vi "Write Data to Log File.vi"(8 "Error In":errorcluster, 10 "queue out":refnum<queue>, 11 "Byte Stream File in":refnum<file>) -> (0 "error out":errorcluster, 3 "Byte Stream File out":refnum<file>)   [LabVIEW 2018]
doc: "Author: Scott Hannahs <sth@magnet.fsu.edu>\nCopyright 2018 Florida State University, All rights reserved."
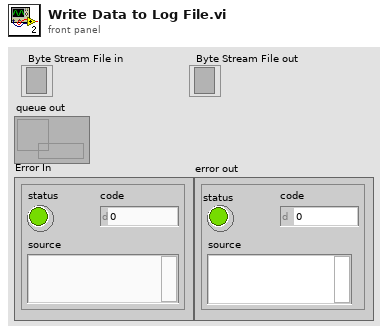
[diagram p1: front panel]
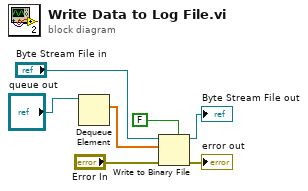
[diagram p0: block diagram]
diagram:
  n1 = Dequeue Element(queue="queue out") -> (element=w1:dbl[])  [unwired: 2 in, 3 out]
  n2 = Write to Binary File(file (use dialog)="Byte Stream File in", data=w1, error in="Error In", 5:FALSE ("prepend array or string size? (T)")) -> (refnum out=→"Byte Stream File out":refnum<file>, error out=→"error out":errorcluster)  [unwired: 2 in, 1 out]
